vi "MPS_Drive_ImonScale.vi"(11 "Drive IMon FFT Mag RMS":dbl) -> (2 "Amps Drive Peak":dbl, 3 "Expected mT Peak":dbl)   [LabVIEW 2021]
uses:
  MPS_global_variables.vi
panel:
  out "Volts per peak amp\nDrive at fDrive":dbl
  out "Drive IMon FFT Mag Peak":dbl
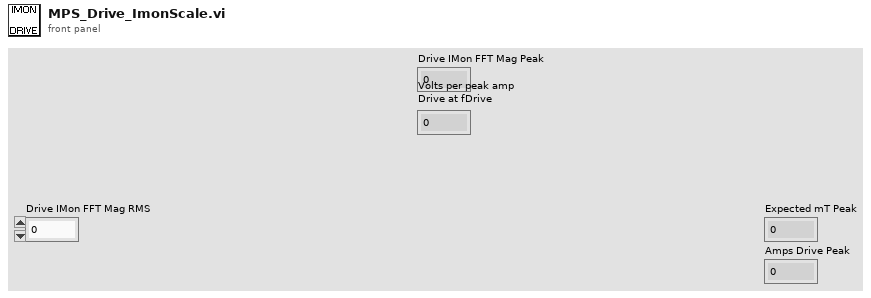
[diagram p1: front panel]
types:
  T1 = cluster{"sample rate":dbl, "Tx freq":dbl, "Tx amp":dbl, "Tx cycles\nSpectroscopy":dbl, "Bias amp":dbl, "Bias freq":dbl, "Receive range":dbl, "Bias Periods\nMagnetometry":dbl, "Tx Freq Division Factor":dbl, "Drive Periods per Bias":dbl, "TX harmonics":dbl[]}
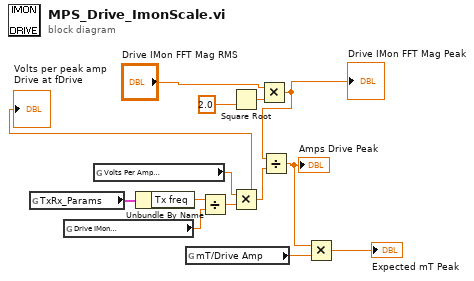
[diagram p0: block diagram]
diagram:
  n1 = global read "MPS_global_variables.vi" "TxRx_Params"() -> (w11:T1)
  n2 = global read "MPS_global_variables.vi" "Drive IMon\nRef Freq"() -> (w9:dbl)
  n3 = global read "MPS_global_variables.vi" "Volts Per Amp\nDrive"() -> (w12:dbl)
  n4 = Unbundle By Name(w11) -> ("Tx freq"=w10:dbl)
  n5 = global read "MPS_global_variables.vi" "mT/Drive Amp"() -> (w5:dbl)
  n6 = Divide(x=w10, y=w9) -> (x/y=w8:dbl)
  n7 = Square Root(x=2.0) -> (sqrt(x)=w4:dbl)
  n8 = Multiply(x=w12, y=w8) -> (x*y=w7:dbl)
  "Volts per peak amp\nDrive at fDrive" <- w7
  n9 = Multiply(x="Drive IMon FFT Mag RMS", y=w4) -> (x*y=w1:dbl)
  "Drive IMon FFT Mag Peak" <- w1
  n10 = Divide(x=w1, y=w7) -> (x/y=w6:dbl)
  "Amps Drive Peak" <- w6
  n11 = Multiply(x=w6, y=w5) -> (x*y=→"Expected mT Peak":dbl)
